vi "close potentiostat.vi"() -> ()   [LabVIEW 2017]
uses:
  C:/Program Files (x86)/Princeton Applied Research/VersaSTAT Development Kit/LabView v2011 Examples/VersaSTATControl.dll
  Program Files (x86)/Princeton Applied Research/VersaSTAT Development Kit/LabView v2011 Examples/VersaSTATControl.dll
  <instrlib>/Princeton potentiostat/Princeton potentiostat.lvlib
panel:
  in  "Potentiostat port":refnum<k24>
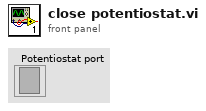
[diagram p1: front panel]
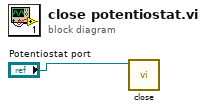
[diagram p0: block diagram]
diagram:
  n1 = call <instrlib>:"close.vi"("reference"="Potentiostat port") -> ()  [unwired: 10 in, 1 out]
